vi "sendRunExperiment.vi"(8 "error in (no error)":errorcluster, 9 "runExperiment.Enum":enum16{"runListOnce", "loopOverList"}(ring), 10 "runExperiment.Array":path[](array[path]), 11 "ExperimentControlEvents in":refnum<class "ExperimentControlEvents.lvclass">) -> (0 "error out":errorcluster, 3 "ExperimentControlEvents out":refnum<class "ExperimentControlEvents.lvclass">)   [LabVIEW 2009, in "Views.lvlib" / "ExperimentControl.lvlib" / "ExperimentControlEvents.lvclass"]
uses:
  ExperimentControlEvents.lvclass
  ExperimentControlEvents.lvclass/ExperimentControlEvents.ctl
  Events/Event.lvclass
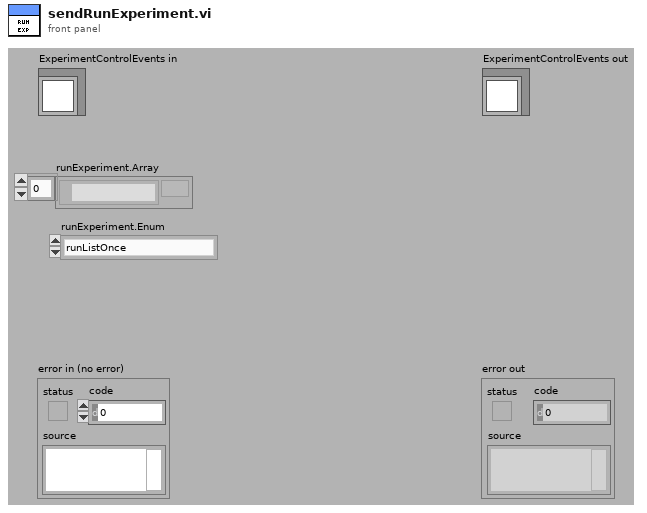
[diagram p1: front panel]
types:
  T1 = enum16{"close", "stopRunning", "runSingleScript", "runExperiment", "runExperimentScript"}
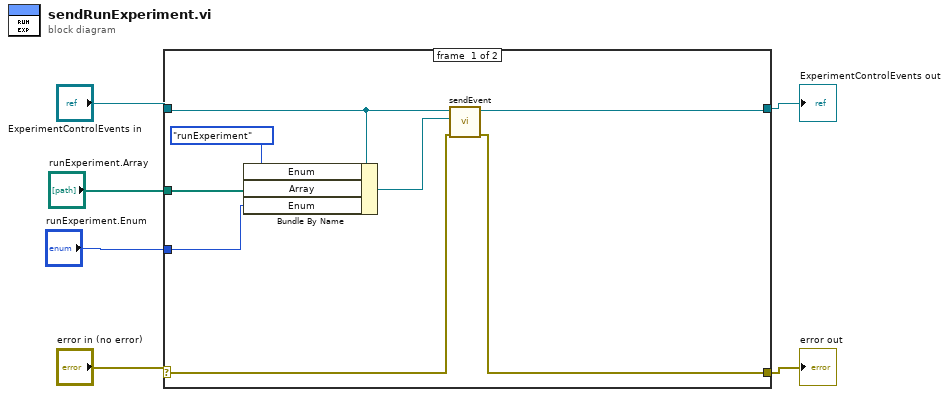
[diagram p0: block diagram]
diagram:
  n1 = case shown="No Error" "error in (no error)" {
    selector: "error in (no error)" -> [w10 w16]
    tunnel: [w9 w16] -> w4
    tunnel: [w14 w15] -> w5
    tunnel: "ExperimentControlEvents in" -> [w13 w15]
    tunnel: "runExperiment.Enum" -> [w8 _]
    tunnel: "runExperiment.Array" -> [w7 _]
    frame #0 {
      n2 = Bundle By Name(cluster=w13, "Enum"=T1."runExperiment", "Array"=w7, "Enum"=w8) -> (w12:refnum<class "ExperimentControlEvents.lvclass">)
      n3 = call "sendEvent.vi"("error in (no error)"=w10, "data"=w12, "Event in"=w13) -> ("error out"=w9:errorcluster, "Event out"=w14:refnum<class "ExperimentControlEvents.lvclass">)  [unwired: 7 in]
    }
    frame #1 {
    }
  }
  "error out" <- w4
  "ExperimentControlEvents out" <- w5
